vi "close.vi"(8 "error in (no error)":errorcluster, 11 "Lesker Pressure in":refnum<class "Lesker Pressure.lvclass">) -> (0 "error out":errorcluster, 3 "Lesker Pressure out":refnum<class "Lesker Pressure.lvclass">)   [LabVIEW 2024, in "Lesker Pressure.lvclass"]
uses:
  Lesker Pressure.lvclass
  Lesker Pressure.lvclass/Lesker Pressure.ctl
  Pressure Monitor.lvclass
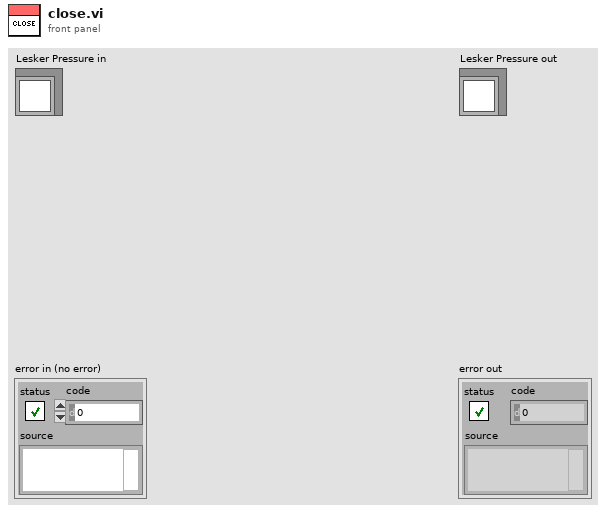
[diagram p1: front panel]
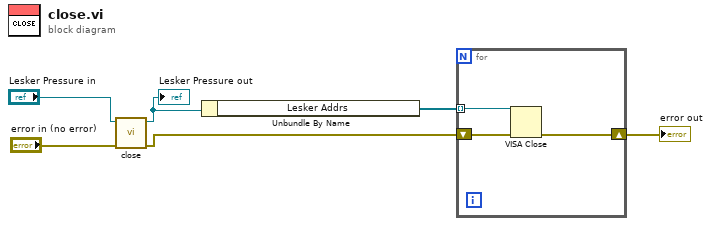
[diagram p0: block diagram]
diagram:
  n1 = call-parent "close.vi"("error in (no error)"="error in (no error)", "Pressure Monitor in"="Lesker Pressure in") -> ("error out"=w2:errorcluster, "Pressure Monitor out"=w4:refnum<class "Lesker Pressure.lvclass">)  [unwired: 8 in]
  "Lesker Pressure out" <- w4
  n2 = Unbundle By Name(w4) -> ("Lesker Addrs"=w3:refnum<visa-resource-name>[])
  n3 = for {
    tunnel: w3 -> [w9] mode=indexing
    shift-right: [w7] -> w1
    shift-left: w2 -> [w8]
    n4 = VISA Close(VISA resource name=w9, error in (no error)=w8) -> (error out=w7:errorcluster)
  }
  "error out" <- w1
